vi "Write Graph Legend Props.vi"(8 "error in (no error)":errorcluster, 10 "Plot Legend Props":T1, 11 "Graph in":refnum<vi>) -> (0 "error out":errorcluster, 3 "Graph":refnum<vi>)   [LabVIEW 2020, in "VolatusGUIEditorCore.lvlib"]
uses:
  VolatusGUIEditorCore.lvlib
  Plot Legend Props.ctl
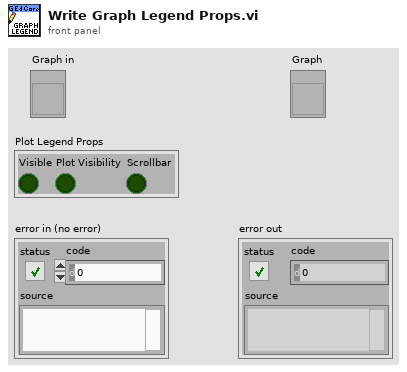
[diagram p1: front panel]
types:
  T1 = typedef "VolatusGUIEditorCore.lvlib/Plot Legend Props.ctl" = cluster{"Visible":bool, "Plot Visibility":bool, "Scrollbar":bool}
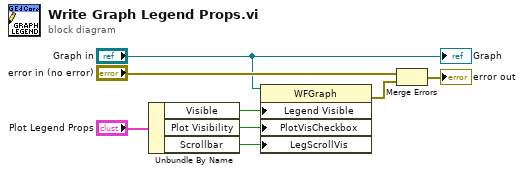
[diagram p0: block diagram]
diagram:
  n1 = Unbundle By Name("Plot Legend Props") -> ("Visible"=w3:bool, "Plot Visibility"=w2:bool, "Scrollbar"=w1:bool)
  n2 = property class="WFGraph"(reference="Graph in", "Legend Visible"=w3, "PlotVisCheckbox"=w2, "LegScrollVis"=w1) -> (error out=w6:errorcluster)  [unwired: 1 in, 1 out]
  n3 = Merge Errors("error in (no error)", w6) -> (→"error out":errorcluster)
  "Graph" <- "Graph in"
